vi "DiffDrivePoseEst_GetEstimatedPosition.vi"(11 "in DiffDrivePoseEstimate":T4={"M_VisionContR"=[], "m_nominal_dT"=0.0, "m_PrevTime_Sec"=0.0, "m_GyroOffset"={"VALUE"=0.0, "COS"=1.0, "SIN"=0.0}, "m_PrevAngle"={"VALUE"=0.0, "COS"=1.0, "SIN"=0.0}, "StartLeftEnc_M"=0.0, "StartRightEnc_M"=0.0, "m_Observer"={"m_P"=[], "m_xHat"=[], "States"=0, "Outputs"=0, "m_ContR"=[], "m_ContQ"=[], "m_SigmasF"=[], "m_dT_Sec"=0.0, "MERWE_SCALED_SIGMA_PTS"={"m_Wm"=[], "States"=0, "Alpha"=0.0, "m_Wc"=[], "Kappa"=0}, "meanFuncX"=refnum, "meanFuncY"=refnum, "residualFuncX"=refnum, "residualFuncY"=refnum, "addFuncX"=refnum, "addFuncXExtra"=variant, "residualFuncYExtra"=variant, "residualFuncXExtra"=variant, "MeanFuncYExtra"=variant, "MeanFuncXExtra"=variant, "Inputs"=0}, "m_latencyCompensator"={"m_pastObserverSnapshots "=[]}} {"m_PrevAngle"."SIN" format="%13.4f"; "m_PrevAngle"."COS" format="%13.4f"; "m_PrevAngle"."VALUE" format="%13.4f"; "m_GyroOffset"."SIN" format="%13.4f"; "m_GyroOffset"."COS" format="%13.4f"; "m_GyroOffset"."VALUE" format="%13.4f"}) -> (3 "Estimated Pose":T1 {"ROTATION"."SIN" format="%13.4f"; "ROTATION"."COS" format="%13.4f"; "ROTATION"."VALUE" format="%13.4f"; "TRANSLATION"."Y" format="%14.3f"; "TRANSLATION"."X" format="%14.3f"})   [LabVIEW 2019, in "Trajectory_Library.lvlib"]
doc: "Gets the pose of the robot at the current time as estimated by the Unscented Kalman Filter.\n \nInputs:\n - DiffDrivePoseEst - System data cluster\n\nOutputs:\n - EstimatedPose - The estimated robot pose in meters."
uses:
  Trajectory_Library.lvlib
  DIFF_DRIVE_POSE_EST.ctl
  <vilib>/Analysis/Matrix/Datatypes/RealMatrix.ctl
  ROTATION2D.ctl
  UNSCENTED_KALMAN_FILTER.ctl
  MERWE_SCALED_SIGMA_PTS.ctl
  CALLBACK_FUNC_TYPE.ctl
  KALMAN_FILTER_LATENCY_COMP.ctl
  OBSERVER_SNAP_LIST_ITEM.ctl
  OBSERVER_SNAPSHOT.ctl
  POSE2D.ctl
  TRANSLATION2D.ctl
  Rotation_CreateAngle.vi
  Translation_Create.vi
  <vilib>/Analysis/Matrix/NI_Matrix.lvlib
panel:
  # "<3, 3>"
  # "<Statess,1>"
  # "<States, States>"
  # "<Inputs, 1>"
  # "<Outputs,  1>"
  # "State Estimate <Statess,1>"
  # "<States, States>"
  # "<States, ?>"
  # "<Statess,  States>"
  # "<Outputs, Outputs>"
  # "<?, 1>"
  # "<?, 1>"
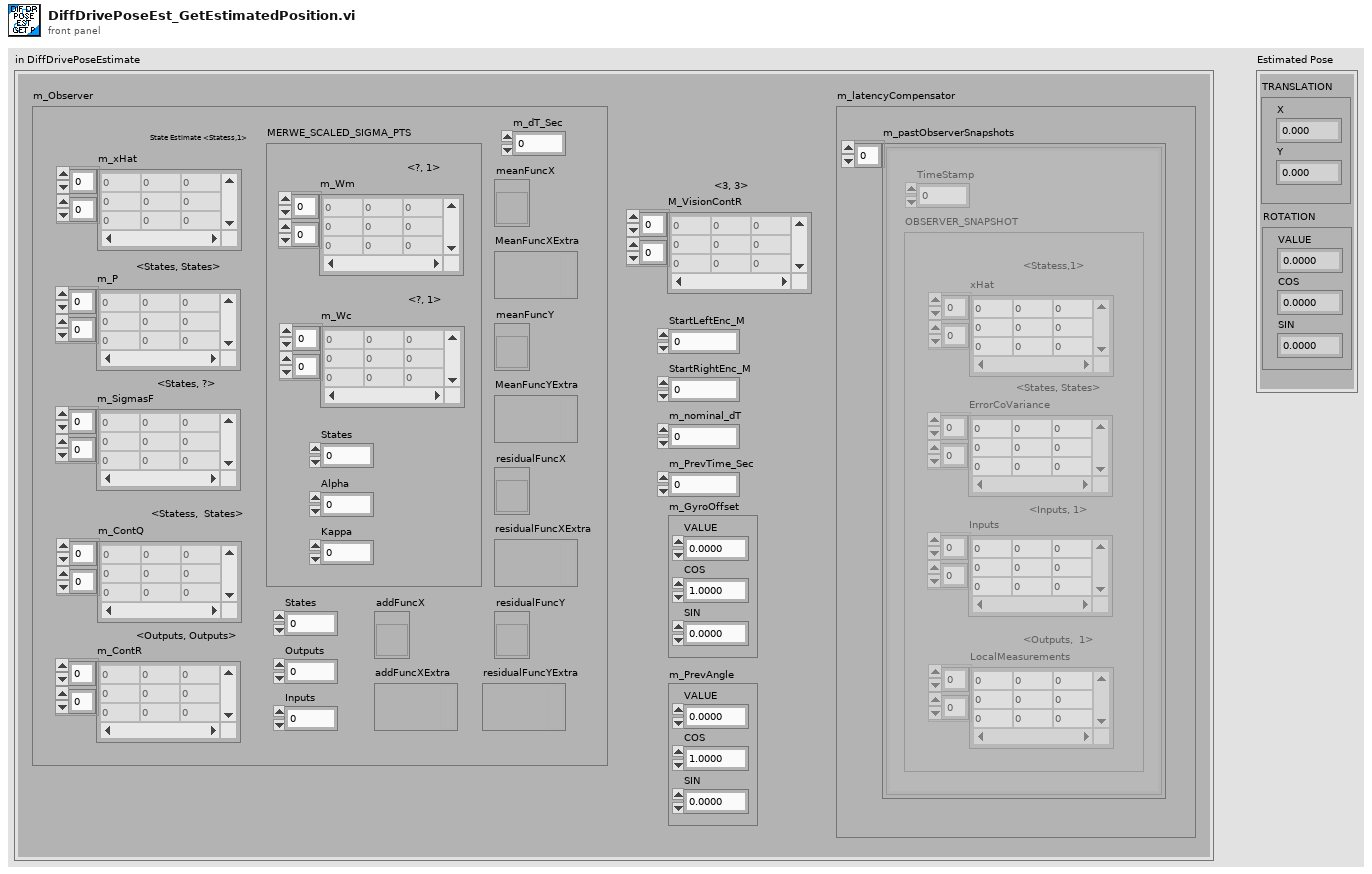
[diagram p1: front panel]
types:
  T1 = typedef "Trajectory_Library.lvlib/POSE2D.ctl" = cluster{"TRANSLATION":T2, "ROTATION":T3}
  T2 = typedef "Trajectory_Library.lvlib/TRANSLATION2D.ctl" = cluster{"X":dbl, "Y":dbl}
  T3 = typedef "Trajectory_Library.lvlib/ROTATION2D.ctl" = cluster{"VALUE":dbl, "COS":dbl, "SIN":dbl}
  T4 = typedef "Trajectory_Library.lvlib/DIFF_DRIVE_POSE_EST.ctl" = cluster{"M_VisionContR":T5, "m_nominal_dT":dbl, "m_PrevTime_Sec":dbl, "m_GyroOffset":T3, "m_PrevAngle":T3, "StartLeftEnc_M":dbl, "StartRightEnc_M":dbl, "m_Observer":T6, "m_latencyCompensator":T9}
  T5 = typedef "NI_Matrix.lvlib/RealMatrix.ctl" = dbl[][]
  T6 = typedef "Trajectory_Library.lvlib/UNSCENTED_KALMAN_FILTER.ctl" = cluster{"m_P":T5, "m_xHat":T5, "States":i32, "Outputs":i32, "m_ContR":T5, "m_ContQ":T5, "m_SigmasF":T5, "m_dT_Sec":dbl, "MERWE_SCALED_SIGMA_PTS":T7, "meanFuncX":T8, "meanFuncY":T8, "residualFuncX":T8, "residualFuncY":T8, "addFuncX":T8, "addFuncXExtra":variant, "residualFuncYExtra":variant, "residualFuncXExtra":variant, "MeanFuncYExtra":variant, "MeanFuncXExtra":variant, "Inputs":i32}
  T7 = typedef "Trajectory_Library.lvlib/MERWE_SCALED_SIGMA_PTS.ctl" = cluster{"m_Wm":T5, "States":i32, "Alpha":dbl, "m_Wc":T5, "Kappa":i32}
  T8 = typedef "Trajectory_Library.lvlib/CALLBACK_FUNC_TYPE.ctl" = refnum<vi>
  T9 = typedef "Trajectory_Library.lvlib/KALMAN_FILTER_LATENCY_COMP.ctl" = cluster{"m_pastObserverSnapshots ":T10[]}
  T10 = typedef "Trajectory_Library.lvlib/OBSERVER_SNAP_LIST_ITEM.ctl" = cluster{"TimeStamp":dbl, "OBSERVER_SNAPSHOT":T11}
  T11 = typedef "Trajectory_Library.lvlib/OBSERVER_SNAPSHOT.ctl" = cluster{"ErrorCoVariance":T5, "xHat":T5, "LocalMeasurements":T5, "Inputs":T5}
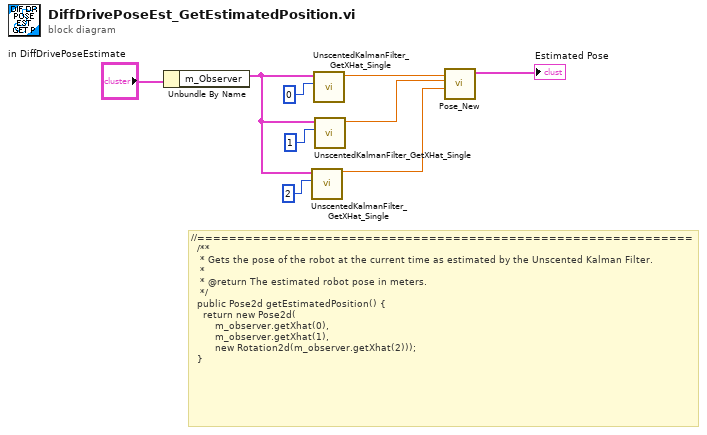
[diagram p0: block diagram]
diagram:
  # "//==============================================================\n  /**\n   * Gets the pose of the robot at the current time as estimated by the Unscented Kalman Filter.\n   *\n   * @return The estimated robot pose in meters.\n   */\n  public Pose2d getEstimatedPosition() {\n    return new Pose2d(\n        m_observer.getXhat(0), \n        m_observer.getXhat(1), \n        new Rotation2d(m_observer.getXhat(2)));\n  }"
  n1 = Unbundle By Name("in DiffDrivePoseEstimate") -> ("m_Observer"=w7:T6)
  n2 = call "UnscentedKalmanFilter_GetXHat_Single.vi"("Row"=2, "in UnscentedKalmanFiilter"=w7) -> ("xHat Value"=w1:dbl)  [unwired: 9 in]
  n3 = call "UnscentedKalmanFilter_GetXHat_Single.vi"("Row"=0, "in UnscentedKalmanFiilter"=w7) -> ("xHat Value"=w3:dbl)  [unwired: 9 in]
  n4 = call "UnscentedKalmanFilter_GetXHat_Single.vi"("Row"=1, "in UnscentedKalmanFiilter"=w7) -> ("xHat Value"=w2:dbl)  [unwired: 9 in]
  n5 = call "Pose_New.vi"("Heading"=w1, "Y"=w2, "X"=w3) -> ("out POSe"=→"Estimated Pose":T1)  [unwired: 8 in]
